vi "onGoing.vi"() -> ()   [LabVIEW 2018]
panel:
  out "Collected Signals":dynamicdata(graph)
  in  "stop (F)":bool
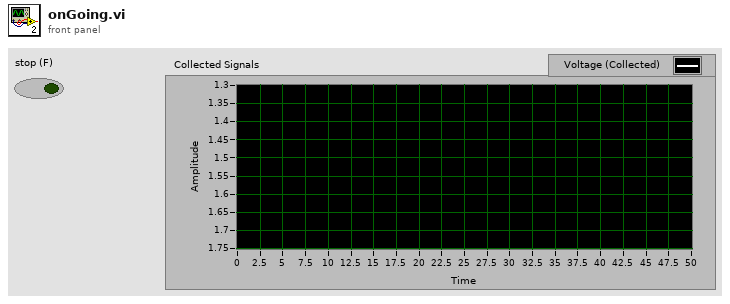
[diagram p1: front panel]
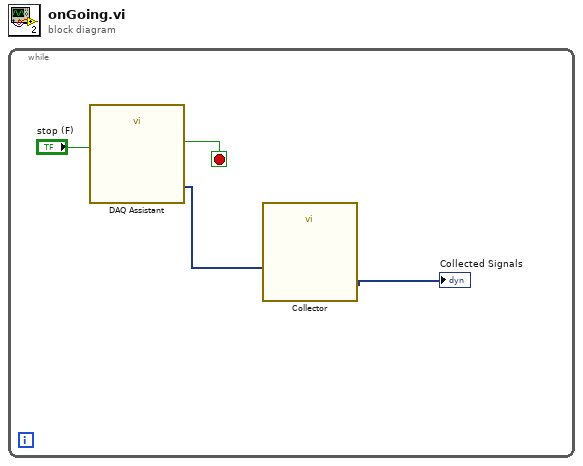
[diagram p0: block diagram]
diagram:
  n1 = while {
    stop <- w3 stop-if-true
    n2 = call "DAQ Assistant"("stop (F)"="stop (F)") -> ("data"=w2:dynamicdata, "stopped"=w3:bool)  [unwired: 15 in, 2 out]
    n3 = call "Collector"("Signals"=w2) -> ("Collected Signals"=→"Collected Signals":dynamicdata)  [unwired: 9 in, 1 out]
  }
